vi "add_DigitalOutputCommand.vi"(4 "Digital Output Command":cluster{"Name":string, "Value":bool}, 5 "msg in":string) -> (2 "msg out":string)   [LabVIEW 2010]
uses:
  Primitives/subs/stringScalar.vi
  Primitives/subs/boolScalar.vi
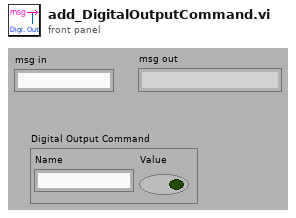
[diagram p1: front panel]
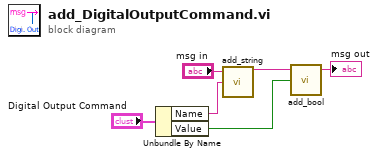
[diagram p0: block diagram]
diagram:
  n1 = Unbundle By Name("Digital Output Command") -> ("Name"=w2:string, "Value"=w1:bool)
  n2 = call-poly "add_string.vi"("String"=w2, "msg in"="msg in") -> ("msg out"=w6:string)  [unwired: 3 in]
  n3 = call-poly "add_bool.vi"("Boolean"=w1, "msg in"=w6) -> ("msg out"=→"msg out":string)  [unwired: 3 in]
